vi "Window Updater.vi"(8 "error in (no error)":errorcluster, 9 "Default Title":string, 10 "Panel":refnum<vi>) -> (0 "error out":errorcluster, 3 "Window Updater out":refnum<class "Window Updater.lvclass">)   [LabVIEW 2023, in "Panel Actor.lvlib" / "Panel.lvlib" / "Window Updater.lvclass"]
doc: "Creates a new Window Updater object\n----\nCopyright: MGI 2017\nAuthor: Derek Trepanier"
uses:
  Window Updater.lvclass
  Window Updater.lvclass/Window Updater.ctl
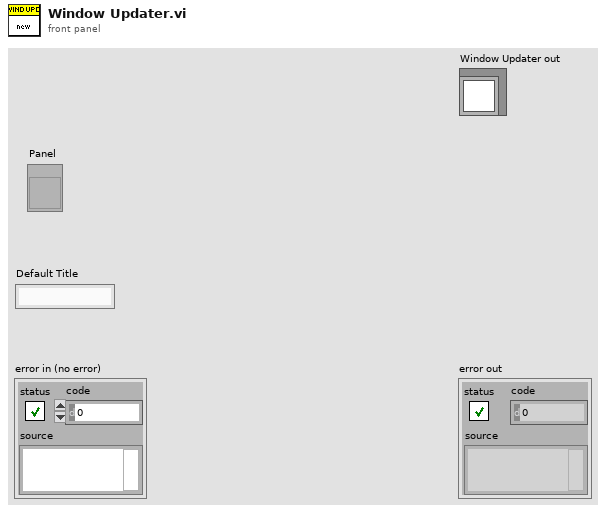
[diagram p1: front panel]
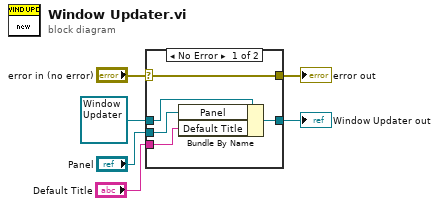
[diagram p0: block diagram]
diagram:
  n1 = case shown="No Error" "error in (no error)" {
    selector: "error in (no error)" -> [w10 w13]
    tunnel: [w10 w13] -> w5
    tunnel: [w9 w12] -> w3
    tunnel: refnum<class "Window Updater.lvclass"> refnum ("Window Updater in") -> [w11 w12]
    tunnel: "Panel" -> [w8 _]
    tunnel: "Default Title" -> [w7 _]
    frame No Error {
      n2 = Bundle By Name(cluster=w11, "Panel"=w8, "Default Title"=w7) -> (w9:refnum<class "Window Updater.lvclass">)
    }
    frame Error {
    }
  }
  "error out" <- w5
  "Window Updater out" <- w3
